vi "ANNsubs_AnalyticalModel.vi"(9 "AngularV":dbl, 11 "linearV":dbl) -> (1 "W R":dbl, 3 "W L":dbl)   [LabVIEW 2017]
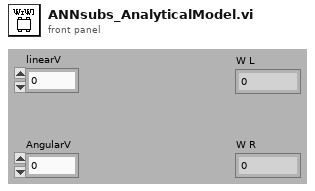
[diagram p1: front panel]
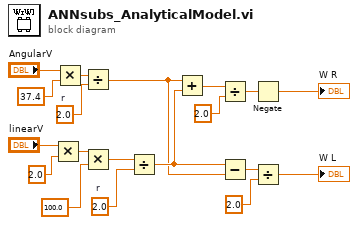
[diagram p0: block diagram]
diagram:
  w5 = 2.0  # r
  w7 = 2.0  # r
  n1 = Multiply(x="linearV", y=2.0) -> (x*y=w14:dbl)
  n2 = Multiply(x="AngularV", y=37.4) -> (x*y=w17:dbl)
  n3 = Divide(x=w17, y=w7) -> (x/y=w2:dbl)
  n4 = Multiply(x=w14, y=100.0) -> (x*y=w6:dbl)
  n5 = Divide(x=w6, y=w5) -> (x/y=w3:dbl)
  n6 = Add(x=w2, y=w3) -> (x+y=w12:dbl)
  n7 = Divide(x=w12, y=2.0) -> (x/y=w4:dbl)
  n8 = Subtract(x=w3, y=w2) -> (x-y=w10:dbl)
  n9 = Negate(x=w4) -> (-x=→"W R":dbl)
  n10 = Divide(x=w10, y=2.0) -> (x/y=→"W L":dbl)
